vi "settingTemplate.vi"() -> ()   [LabVIEW 2017]
panel:
  in  "退出":bool
  in  "保存":bool
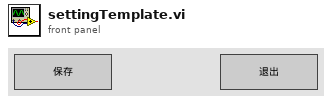
[diagram p1: front panel]
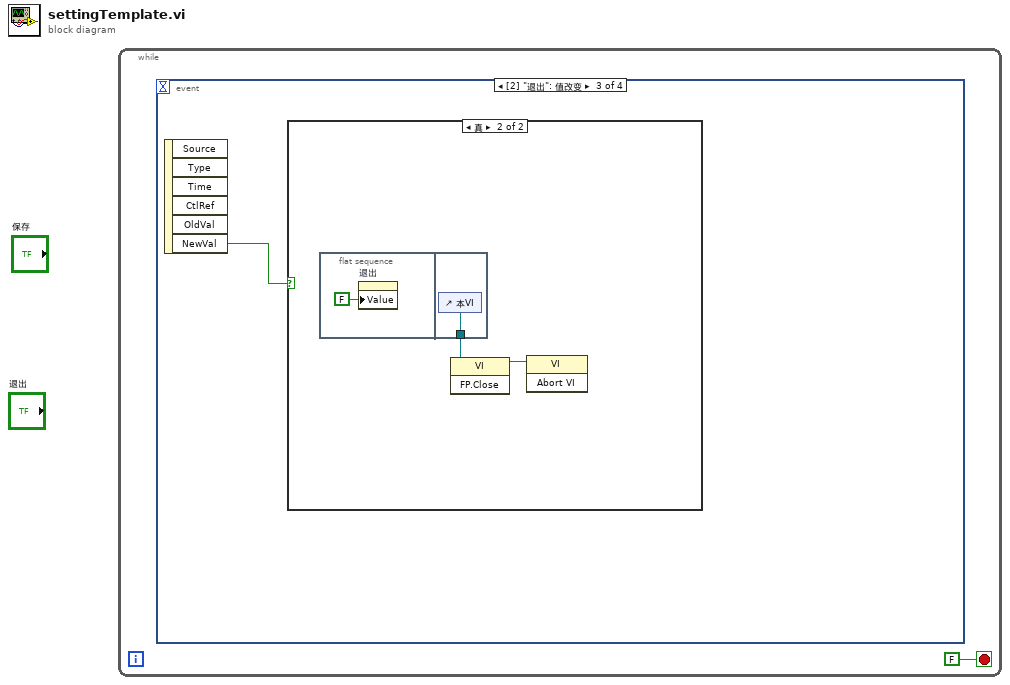
[diagram p0: block diagram]
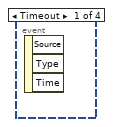
[diagram p2: hidden frame]
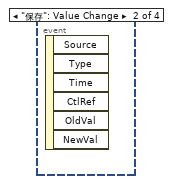
[diagram p3: hidden frame]
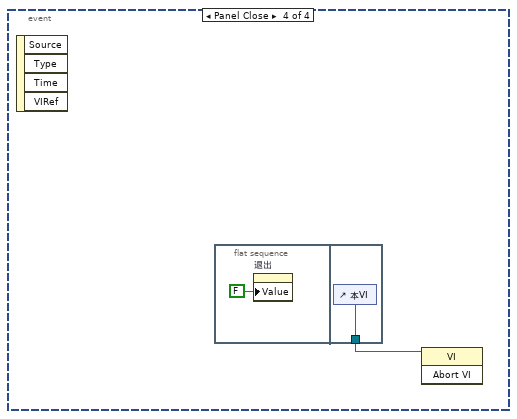
[diagram p5: hidden frame]
diagram:
  n1 = while {
    stop <- FALSE stop-if-true
    n2 = event shown="[2] \"退出\": 值改变" {
      selector: _ -> [_ _ _ _]
      dyn-events: _ -> [_ _ _ _]
      timeout: _ -> [_ _ _ _]
      event Timeout {
        n3 = event-data() -> ()  [unwired: 1 in, 3 out]
      }
      event "保存": Value Change {
        n4 = event-data() -> ()  [unwired: 1 in, 6 out]
      }
      event "退出": Value Change {
        n5 = event-data() -> ("NewVal"=w2:bool)  [unwired: 1 in, 5 out]
        n6 = case shown="真" w2 {
          frame False {
          }
          frame True {
            n7 = flat-sequence {
              tunnel: [w6] -> w4
              frame #0 {
                n8 = property on="退出" class="Bool (严格)"("Value"=FALSE ("退出")) -> ()  [unwired: 2 in, 2 out]
              }
              frame #1 {
                n9 = control-ref of="本VI"() -> (w6:refnum<vi>)
              }
            }
            n10 = invoke class="VI" method="FP.Close"(reference=w4) -> (reference out=w3:refnum<vi>)  [unwired: 2 in, 2 out]
            n11 = invoke class="VI" method="Abort VI"(reference=w3) -> ()  [unwired: 2 in, 3 out]
          }
        }
      }
      event Panel Close {
        n12 = event-data() -> ()  [unwired: 1 in, 4 out]
        n13 = flat-sequence {
          tunnel: [w9] -> w7
          frame #0 {
            n14 = property on="退出" class="Bool (严格)"("Value"=FALSE ("退出")) -> ()  [unwired: 2 in, 2 out]
          }
          frame #1 {
            n15 = control-ref of="本VI"() -> (w9:refnum<vi>)
          }
        }
        n16 = invoke class="VI" method="Abort VI"(reference=w7) -> ()  [unwired: 2 in, 3 out]
      }
    }
  }
